vi "Create_Filename.vi"(3 "error in":errorcluster, 4 "Path in":path, 5 "Base name":string) -> (0 "error out":errorcluster, 1 "Path out":path, 2 "Output filename":string)   [LabVIEW 2015]
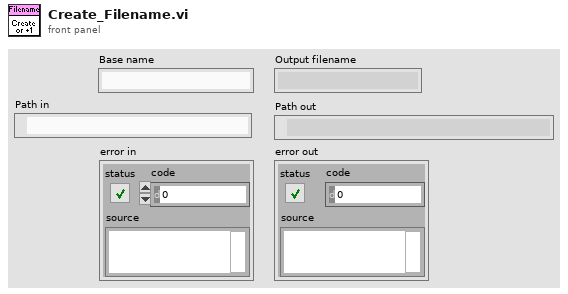
[diagram p1: front panel]
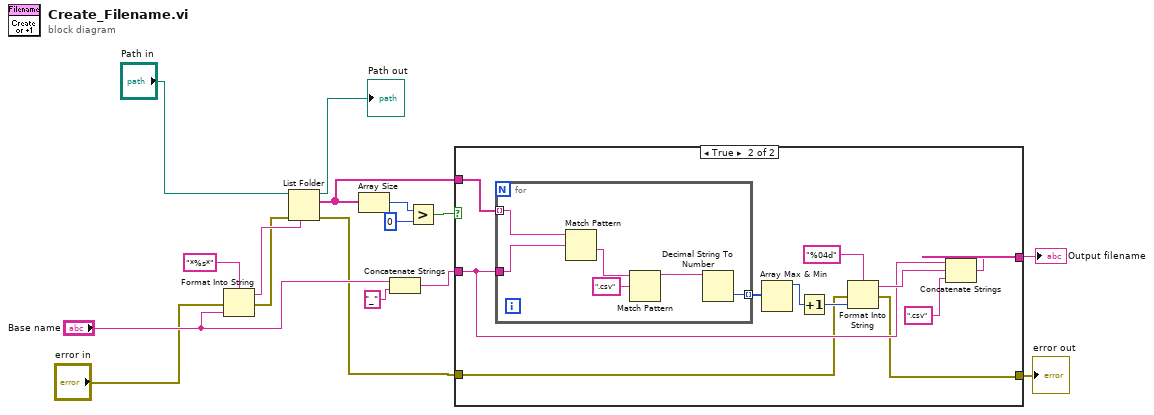
[diagram p0: block diagram]
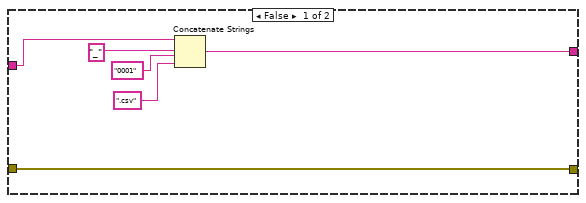
[diagram p2: hidden frame]
diagram:
  n1 = Format Into String(format string="*%s*", error in="error in", "Base name") -> (resulting string=w7:string, error out=w6:errorcluster)  [unwired: 1 in]
  n2 = List Folder(path="Path in", pattern=w7, error in=w6) -> (path out=→"Path out":path, filenames=w13:string[], error out=w5:errorcluster)  [unwired: 1 in, 1 out]
  n3 = Array Size(array=w13) -> (size(s)=w14:i32)
  n4 = Concatenate Strings("Base name", "_" ("string")) -> (w12:string)
  n5 = Greater?(x=w14, y=0) -> (0:w16:bool)
  n6 = case shown="True" w16 {
    tunnel: w12 -> [w22 w28]
    tunnel: w13 -> [_ w30]
    tunnel: [w18 w25] -> w10
    tunnel: w5 -> [w17 w27]
    tunnel: [w17 w26] -> w3
    frame False {
      n7 = Concatenate Strings "Concatenate Strings"(w22, "_" ("string"), "0001" ("string"), ".csv" ("string")) -> (w18:string)
    }
    frame True {
      n8 = for {
        tunnel: w30 -> [w39] mode=indexing
        tunnel: w28 -> [w38]
        tunnel: [w34] -> w33 mode=indexing
        n9 = Match Pattern(string=w39, regular expression=w38) -> (after substring=w37:string)  [unwired: 1 in, 3 out]
        n10 = Match Pattern(string=w37, regular expression=".csv") -> (before substring=w35:string)  [unwired: 1 in, 3 out]
        n11 = Decimal String To Number(string=w35) -> (number=w34:i32)  [unwired: 2 in, 1 out]
      }
      n12 = Array Max & Min(array=w33) -> (max value=w32:i32)  [unwired: 3 out]
      n13 = Increment(x=w32) -> (x+1=w31:i32)
      n14 = Format Into String(format string="%04d", error in=w27, w31) -> (resulting string=w29:string, error out=w26:errorcluster)  [unwired: 1 in]
      n15 = Concatenate Strings(w28, w29, ".csv" ("string")) -> (w25:string)
    }
  }
  "Output filename" <- w10
  "error out" <- w3
